vi "read_couter.vi"(7 "Enum":T1(ring), 8 "error in":errorcluster, 10 "counter":tag) -> (0 "error out":errorcluster, 2 "data":dbl format="%0.2f")   [LabVIEW 2015]
uses:
  <vilib>/DAQmx/read.llb/DAQmx Read (Counter DBL 1Chan 1Samp).vi
  <vilib>/DAQmx/create/channels.llb/DAQmx Create Channel (CI-Position-Angular Encoder).vi
  <vilib>/DAQmx/miscellaneous.llb/DAQmx Fill In Error Info.vi
panel:
  out "error out 2":errorcluster
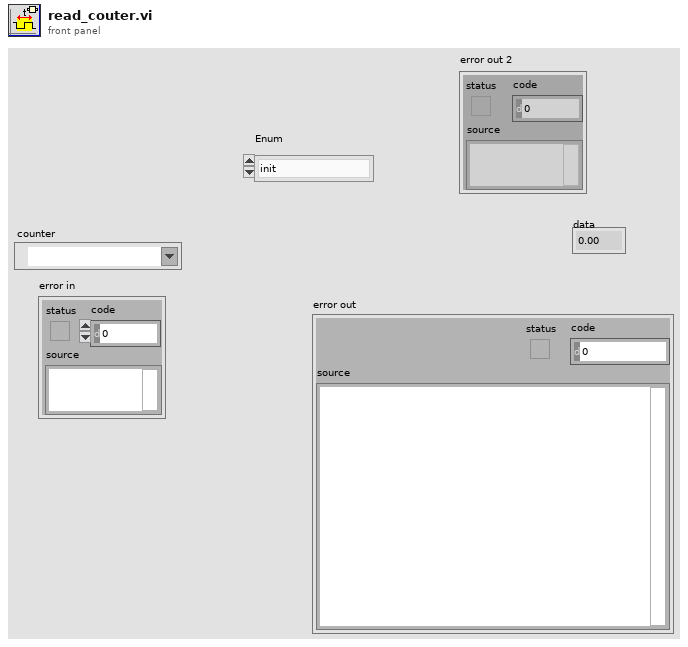
[diagram p1: front panel]
types:
  T1 = enum16{"init", "config", "start", "read", "stop"}
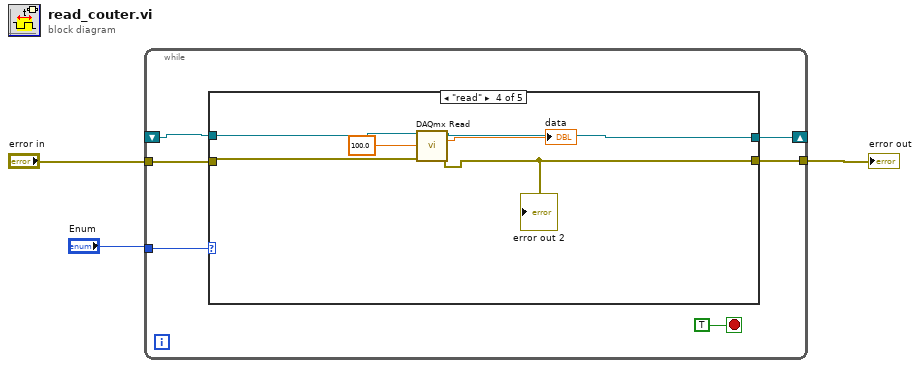
[diagram p0: block diagram]
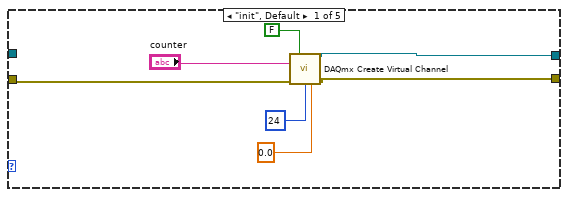
[diagram p2: hidden frame]
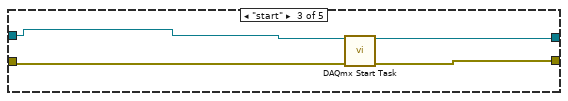
[diagram p4: hidden frame]
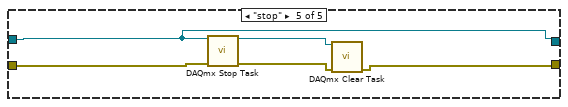
[diagram p5: hidden frame]
diagram:
  n1 = while {
    tunnel: "Enum" -> [w8]
    shift-right: [w7] -> _
    shift-left: _ -> [w6]
    tunnel: "error in" -> [w5]
    tunnel: [w4] -> w1
    stop <- TRUE stop-if-true
    n2 = case shown="\"read\"" w8 {
      tunnel: [w16 w18 w22 w26 w29] -> w7
      tunnel: w6 -> [_ w18 w20 w28 w29]
      tunnel: w5 -> [w14 w17 w19 w27 w33]
      tunnel: [w13 w17 w21 w25 w32] -> w4
      frame "init", Default {
        n3 = call-poly <vilib>:"DAQmx Create Virtual Channel.vi"("z index enable"=FALSE, "counter"="counter", "error in"=w14, "pulses per revolution"=u32 24, "initial angle"=0.0) -> ("task out"=w16:refnum<k21>, "error out"=w13:errorcluster)  [unwired: 9 in]
      }
      frame "config" {
      }
      frame "start" {
        n4 = call <vilib>:"DAQmx Start Task.vi"("task/channels in"=w20, "error in"=w19) -> ("task out"=w22:refnum<k21>, "error out"=w21:errorcluster)  [unwired: 12 in]
      }
      frame "read" {
        n5 = call-poly <vilib>:"DAQmx Read.vi"("task/channels in"=w28, "timeout"=100.0, "error in"=w27) -> ("task out"=w26:refnum<k21>, "data"=→"data":dbl, "error out"=w25:errorcluster)  [unwired: 10 in]
        "error out 2" <- w25
      }
      frame "stop" {
        n6 = call <vilib>:"DAQmx Stop Task.vi"("task/channels in"=w29, "error in"=w33) -> ("task out"=w31:refnum<k21>, "error out"=w30:errorcluster)  [unwired: 12 in]
        n7 = call <vilib>:"DAQmx Clear Task.vi"("task in"=w31, "error in"=w30) -> ("error out"=w32:errorcluster)  [unwired: 13 in]
      }
    }
  }
  "error out" <- w1
